vi "Untitled 5 (SubVI).vi"(10 "time_1":u32, 11 "millisecond timer value":u32) -> (3 "Boolean":bool)   [LabVIEW 2015]
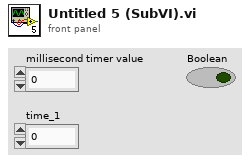
[diagram p1: front panel]
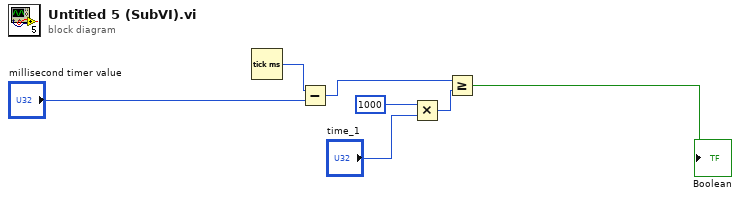
[diagram p0: block diagram]
diagram:
  n1 = Tick Count (ms)() -> (millisecond timer value=w1:u32)
  n2 = Subtract(x=w1, y="millisecond timer value") -> (x-y=w3:u32)
  n3 = Multiply(x=u32 1000 ("y"), y="time_1") -> (x*y=w7:u32)
  n4 = Greater Or Equal?(x=w3, y=w7) -> (x >= y?=→"Boolean":bool)
